vi "CvrtCell2Data.vi"(8 "error in (no error)":errorcluster, 9 "ge_HdrNames":T1, 10 "Item Name":string, 11 "Current in":refnum<class "Current.lvclass">) -> (0 "error out":errorcluster, 3 "Current out":refnum<class "Current.lvclass">)   [LabVIEW 2018, in "Measurement Channels.lvlib" / "Current.lvclass"]
uses:
  Current.lvclass
  Common/Controls/HeaderNames.ctl
  SubVIs Table/Custom Ctls Table/ge_ColType.ctl
  Current.lvclass/Current.ctl
  Class Channel/Channel.lvclass
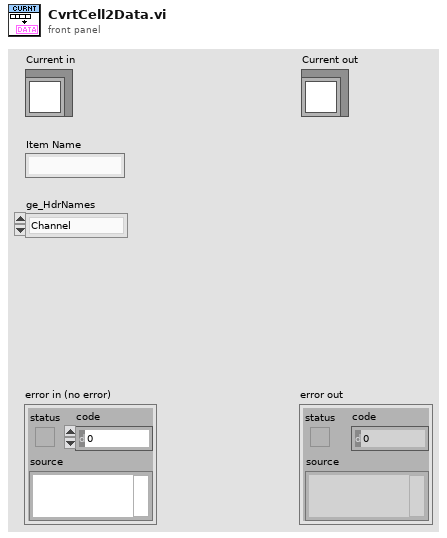
[diagram p1: front panel]
types:
  T1 = typedef "HeaderNames.ctl" = enum16{"Channel", "Device", "Spacer", "Description", "MB", "Range", "Terminal", "Coupling", "Thresh (V)", "Pulse/Rev", "Slope", "Min EU", "Min RPM", "mV/EU", "Iex", "Temp Units", "Type", "CJC Src", "CJC Val", "Ro", "Wire Cfg", "Strain Mode", "Vex", "Bridge Type", "GF", "Gauge Res", "Poisson", "Lead Res", "Init Strain", "GAF", "Scale", "Offset", "Unit (EU)", "dB?", "dB Ref", "Cal Mag", "Cal Units", "Max Temp", "Min Temp", "Max Strain", "Min Strain"}
  T2 = typedef "ge_ColType.ctl" = enum16{"Volts", "Amps", "Ohms", "TermCfg", "WireCfg", "Coup", "Slope", "Iex", "CalUnits", "ThrmUnits", "ThrmType", "CJCSrc", "BrdgType", "Strn Mode", "RTDType"}
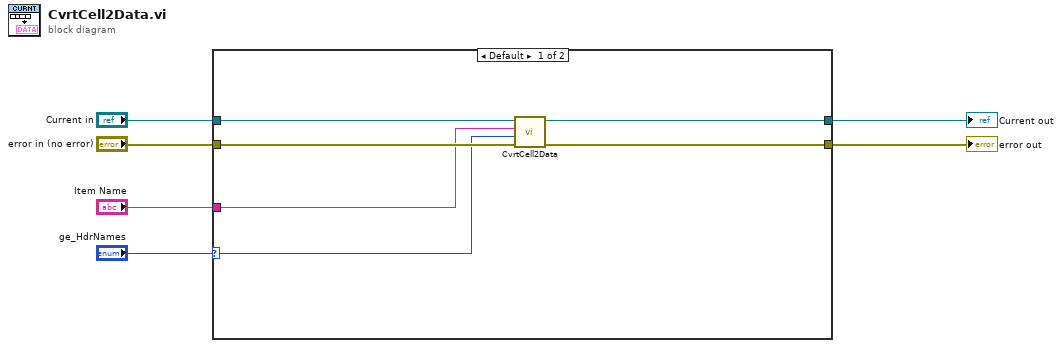
[diagram p0: block diagram]
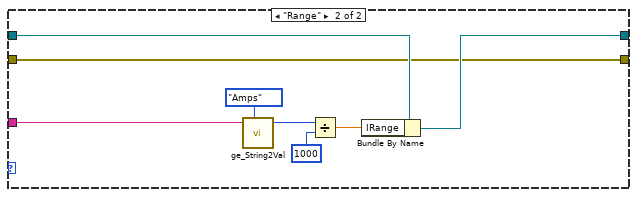
[diagram p2: hidden frame]
diagram:
  n1 = case shown="Default" "ge_HdrNames" {
    selector: "ge_HdrNames" -> [w7 _]
    tunnel: "Current in" -> [w12 w20]
    tunnel: "error in (no error)" -> [w11 w18]
    tunnel: [w10 w19] -> w4
    tunnel: [w9 w18] -> w3
    tunnel: "Item Name" -> [w8 w16]
    frame Default {
      n2 = call-parent "CvrtCell2Data.vi"("error in (no error)"=w11, "Header Names"=w7, "Item Name"=w8, "Channel in"=w12) -> ("error out"=w9:errorcluster, "Channel out"=w10:refnum<class "Current.lvclass">)  [unwired: 6 in]
    }
    frame "Range" {
      n3 = call "ge_String2Val.vi"("String"=w16, "ColType"=ge_ColType."Amps") -> ("Value"=w14:u16)  [unwired: 4 in, 1 out]
      n4 = Divide(x=w14, y=1000) -> (x/y=w13:dbl)
      n5 = Bundle By Name(cluster=w20, "IRange"=w13) -> (w19:refnum<class "Current.lvclass">)
    }
  }
  "error out" <- w3
  "Current out" <- w4
